vi "List Child Class Paths.vi"(8 "error in":errorcluster, 11 "[Class Objects]":refnum<class>[](array[class])) -> (0 "error out":errorcluster, 2 "Child Class Names":string[](array[string]), 3 "Child Class Paths":path[](array[path]))   [LabVIEW 2024, in "Thermal Chamber.lvlib"]
doc: "Returns the names and paths for all classes contained in <B>[Class Objects]</B>, excluding any classes that start with an underscore."
uses:
  Thermal Chamber.lvlib
  <userlib>/_OpenG.lib/file/file.llb/Strip Path Extension - String__ogtk.vi
  <userlib>/_OpenG.lib/file/file.llb/openg_file.lvlib
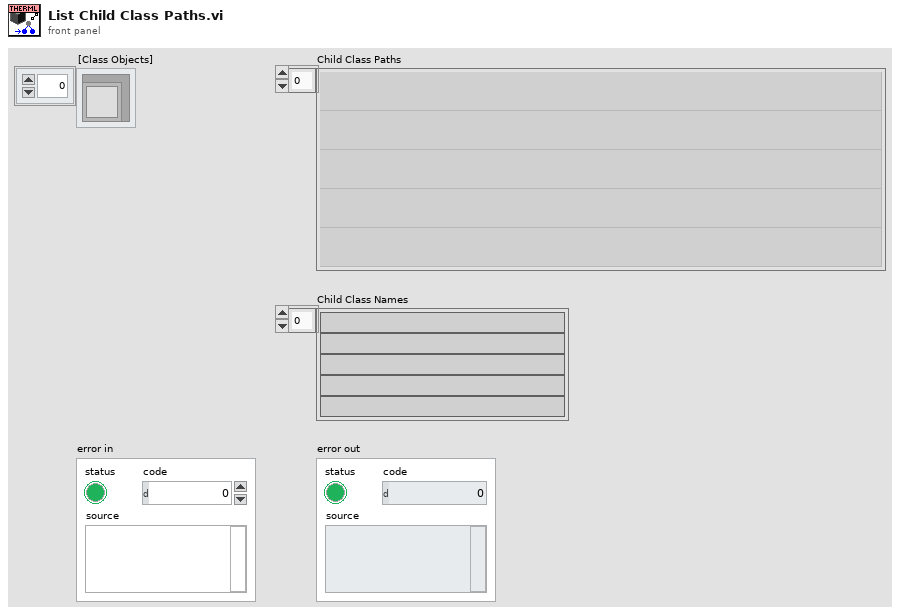
[diagram p1: front panel]
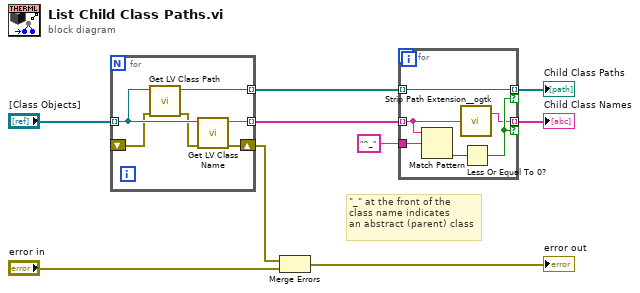
[diagram p0: block diagram]
diagram:
  # "\"_\" at the front of the\nclass name indicates\nan abstract (parent) class"
  n1 = for {
    tunnel: "[Class Objects]" -> [w15] mode=indexing
    tunnel: [w14] -> w7 mode=indexing
    tunnel: [w13] -> w8 mode=indexing
    shift-right: [w12] -> w3
    shift-left: _ -> [w10]
    n2 = call <vilib>:"Get LV Class Path.vi"("error in (no error)"=w10, "object"=w15) -> ("error out"=w11:errorcluster, "class path"=w14:path)  [unwired: 8 in]
    n3 = call <vilib>:"Get LV Class Name.vi"("error in (no error)"=w11, "object"=w15) -> ("error out"=w12:errorcluster, "class name"=w13:string)  [unwired: 8 in]
  }
  n4 = Merge Errors(w3, "error in") -> (→"error out":errorcluster)
  n5 = for {
    tunnel: w8 -> [w16] mode=indexing
    tunnel: "^_" ("regular expression") -> [w21]
    tunnel: [w17] -> w5 mode=indexing if=w19
    tunnel: w7 -> [w18] mode=indexing
    tunnel: [w18] -> w6 mode=indexing if=w19
    n6 = Match Pattern(string=w16, regular expression=w21) -> (offset past match=w20:i32)  [unwired: 1 in, 3 out]
    n7 = call-poly <userlib>:"Strip Path Extension__ogtk.vi"("path"=w16) -> ("root"=w17:string)  [unwired: 1 out]
    n8 = Less Or Equal To 0?(x=w20) -> (x <= 0?=w19:bool)
  }
  "Child Class Paths" <- w6
  "Child Class Names" <- w5
